vi "attribute_read_int64.vi"(5 "Repeated Capability":string, 7 "Attribute":T1={"Identifier"="", "Descriptive name"="", "Data Type"=enum."Integer 32", "Command"="", "Access"=2, "Range Table"="", "Read Callback"="", "Write Callback"="", "Range Callback"="", "Check Callback"="", "Rngtable Callback"="", "Coerce Callback"="", "Supported Models"="", "Instrument Options"="", "Repeated Capabilities"="", "Check Status Callback"="", "Index"=0, "Flag: OPC Wait"=FALSE, "Flag: Dont check status"=FALSE, "Flag: Cache Only"=FALSE} {"Access" items=["Read Only", "Write Only", "Read/Write"]}, 8 "error in":errorcluster, 11 "VISA resource name":refnum<visa-resource-name>) -> (0 "error out":errorcluster, 2 "int64 out":i64, 3 "VISA resource name out":refnum<visa-resource-name>)   [LabVIEW 2014, in "rszvl_rsidr_core.lvlib"]
uses:
  rszvl_rsidr_core.lvlib
  type_Attribute.ctl
  type_Attribute_Data_Type.ctl
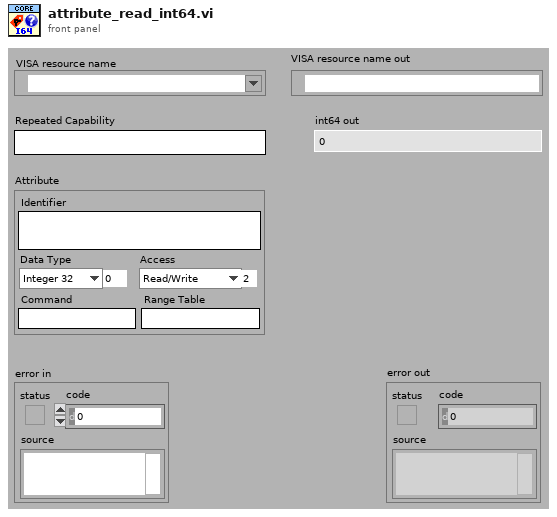
[diagram p1: front panel]
types:
  T1 = typedef "rszvl_rsidr_core.lvlib/type_Attribute.ctl" = cluster{"Identifier":string, "Descriptive name":string, "Data Type":T2, "Command":string, "Access":u16, "Range Table":string, "Read Callback":string, "Write Callback":string, "Range Callback":string, "Check Callback":string, "Rngtable Callback":string, "Coerce Callback":string, "Supported Models":string, "Instrument Options":string, "Repeated Capabilities":string, "Check Status Callback":string, "Index":i32, "Flag: OPC Wait":bool, "Flag: Dont check status":bool, "Flag: Cache Only":bool}
  T2 = typedef "rszvl_rsidr_core.lvlib/type_Attribute_Data_Type.ctl" = enum16{"Integer 32", "Double", "String", "Boolean", "None", "Integer 64"}
  T3 = typedef "rszvl_rsidr_core.lvlib/type_Session_Data.ctl" = cluster{"Instr type":string, "Instr type for err. msg.":string, "Installed Options":string[], "OPC Timeout":i32, "Query Instrument Status":bool, "Check Range":bool, "Check Options":bool, "Add LF to Write":bool, "Simulate":bool, "Logging":bool, "Logging params":variant, "Interface Type":enum16{"Unknown", "GPIB", "VXI", "GPIB_VXI", "ASRL", "PXI", "TCPIP", "USB", "SOCKET"}, "Fast Sweep":i32, "AdditionalFlags":i32, "WaitBeforeWrite":i32, "WaitBeforeRead":i32, "BinDataChunkSize":i64}
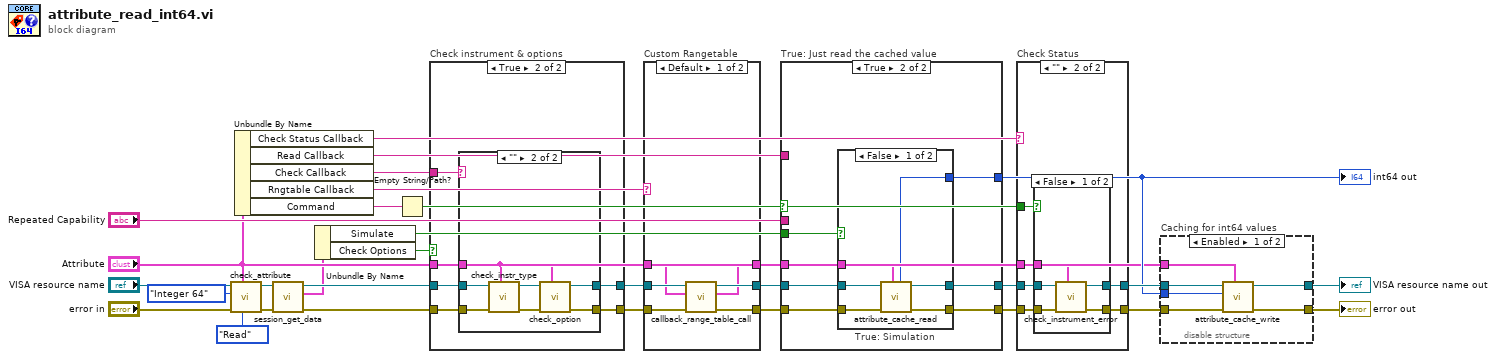
[diagram p0: block diagram]
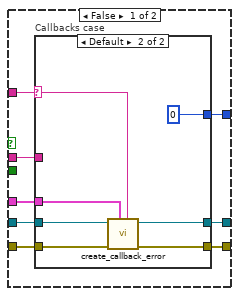
[diagram p2: hidden frame]
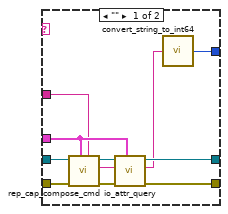
[diagram p3: hidden frame]
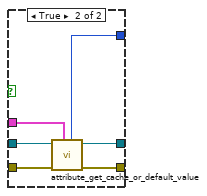
[diagram p4: hidden frame]
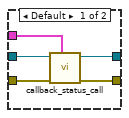
[diagram p6: hidden frame]
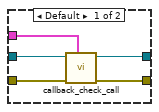
[diagram p9: hidden frame]
diagram:
  n1 = call "check_attribute.vi"("Access"=enum16{"Read", "Write"}."Read", "Attribute"="Attribute", "error in"="error in", "Data Type"=type_Attribute_Data_Type."Integer 64", "VISA resource name"="VISA resource name") -> ("error out"=w17:errorcluster, "VISA resource name out"=w18:refnum<visa-resource-name>)  [unwired: 5 in]
  n2 = Unbundle By Name("Attribute") -> ("Check Status Callback"=w19:string, "Read Callback"=w20:string, "Check Callback"=w9:string, "Rngtable Callback"=w10:string, "Command"=w5:string)
  n3 = call "session_get_data.vi"("error in"=w17, "VISA resource name"=w18) -> ("error out"=w3:errorcluster, "Session User Data out"=w1:T3, "VISA resource name out"=w16:refnum<visa-resource-name>)  [unwired: 7 in]
  n4 = Unbundle By Name(w1) -> ("Simulate"=w2:bool, "Check Options"=w15:bool)
  n5 = Empty String/Path?(string/path=w5) -> (empty?=w28:bool)
  n6 = case "Check instrument & options" shown="True" w15 {
    tunnel: [w33 w39] -> w14
    tunnel: [w32 w38] -> w13
    tunnel: w9 -> [_ w37]
    tunnel: w3 -> [w32 w36]
    tunnel: w16 -> [w33 w35]
    tunnel: "Attribute" -> [_ w34]
    frame False {
    }
    frame True {
      n7 = case shown="\"\"" w37 {
        tunnel: [w43 w49] -> w39
        tunnel: [w41 w48] -> w38
        tunnel: w36 -> [w42 w47]
        tunnel: w35 -> [w44 w46]
        tunnel: w34 -> [w40 w45]
        frame Default {
          n8 = call "callback_check_call.vi"("Attribute"=w40, "error in"=w42, "VISA resource name"=w44) -> ("error out"=w41:errorcluster, "VISA resource name out"=w43:refnum<visa-resource-name>)  [unwired: 7 in]
        }
        frame "" {
          n9 = call "check_instr_type.vi"("Attribute"=w45, "error in"=w47, "VISA resource name"=w46) -> ("error out"=w51:errorcluster, "VISA resource name out"=w50:refnum<visa-resource-name>)  [unwired: 6 in, 1 out]
          n10 = call "check_option.vi"("Attribute"=w45, "error in"=w51, "VISA resource name"=w50) -> ("error out"=w48:errorcluster, "VISA resource name out"=w49:refnum<visa-resource-name>)  [unwired: 7 in]
        }
      }
    }
  }
  n11 = case "Custom Rangetable" shown="Default" w10 {
    tunnel: w14 -> [w57 w60]
    tunnel: w13 -> [w54 w59]
    tunnel: [w56 w60] -> w12
    tunnel: [w55 w59] -> w11
    tunnel: "Attribute" -> [w53 w58]
    tunnel: [w52 w58] -> w8
    frame Default {
      n12 = call "callback_range_table_call.vi"("error in"=w54, "Attribute in"=w53, "VISA resource name"=w57) -> ("error out"=w55:errorcluster, "Attribute out"=w52:T1, "VISA resource name out"=w56:refnum<visa-resource-name>)  [unwired: 6 in]
    }
    frame "" {
    }
  }
  n13 = case "True: Just read the cached value" shown="True" w28 {
    tunnel: "Repeated Capability" -> [w68 _]
    tunnel: [w67 w91] -> w22
    tunnel: [w66 w90] -> w21
    tunnel: [w65 w88] -> w23
    tunnel: w20 -> [w64 _]
    tunnel: w12 -> [w63 w93]
    tunnel: w11 -> [w62 w92]
    tunnel: w8 -> [w61 w89]
    tunnel: w2 -> [_ w87]
    frame False {
      n14 = case "Callbacks case" shown="Default" w64 {
        selector: w64 -> [_ w80]
        tunnel: w63 -> [w79 w84]
        tunnel: w62 -> [w78 w85]
        tunnel: w68 -> [w72 _]
        tunnel: [w71 w82] -> w66
        tunnel: [w69 w83] -> w67
        tunnel: [w77 i64 0 ("int64 value out")] -> w65
        tunnel: w61 -> [w73 w81]
        frame "" {
          n15 = call "rep_cap_compose_cmd.vi"("Repeated Capability"=w72, "Attribute"=w73, "error in"=w78, "VISA resource name"=w79) -> ("error out"=w76:errorcluster, "Command out"=w74:string, "VISA resource name out"=w75:refnum<visa-resource-name>)  [unwired: 5 in]
          n16 = call "io_attr_query.vi"("Attribute"=w73, "error in"=w76, "write buffer"=w74, "VISA resource name"=w75) -> ("error out"=w69:errorcluster, "read buffer"=w70:string, "VISA resource name out"=w71:refnum<visa-resource-name>)  [unwired: 5 in]
          n17 = call "convert_string_to_int64.vi"("String in"=w70) -> ("int64 value out"=w77:i64)  [unwired: 4 in]
        }
        frame Default {
          n18 = call "create_callback_error.vi"("Callback Name"=w80, "Attribute"=w81, "error in"=w85, "VISA resource name"=w84) -> ("error out"=w83:errorcluster, "VISA resource name out"=w82:refnum<visa-resource-name>)  [unwired: 6 in]
        }
      }
    }
    frame True {
      n19 = case "True: Simulation" shown="False" w87 {
        tunnel: w92 -> [w99 w105]
        tunnel: w93 -> [w98 w104]
        tunnel: w89 -> [w97 w101]
        tunnel: [w96 w103] -> w91
        tunnel: [w95 w102] -> w90
        tunnel: [w94 w100] -> w88
        frame False {
          n20 = call "attribute_cache_read.vi"("Attribute"=w97, "error in"=w99, "VISA resource name"=w98) -> ("error out"=w96:errorcluster, "VISA resource name out"=w95:refnum<visa-resource-name>, "Integer 64 out"=w94:i64)  [unwired: 1 in, 5 out]
        }
        frame True {
          n21 = call "attribute_get_cache_or_default_value.vi"("Attribute"=w101, "error in"=w105, "VISA resource name"=w104) -> ("error out"=w103:errorcluster, "VISA resource name out"=w102:refnum<visa-resource-name>, "Integer 64 out"=w100:i64)  [unwired: 1 in, 5 out]
        }
      }
    }
  }
  "int64 out" <- w23
  n22 = case "Check Status" shown="\"\"" w19 {
    tunnel: w22 -> [w110 w114]
    tunnel: [w109 w113] -> w27
    tunnel: [w108 w115] -> w26
    tunnel: w21 -> [w107 w116]
    tunnel: w8 -> [w106 w112]
    tunnel: w28 -> [_ w111]
    frame Default {
      n23 = call "callback_status_call.vi"("Attribute"=w106, "error in"=w110, "VISA resource name"=w107) -> ("error out"=w109:errorcluster, "VISA resource name out"=w108:refnum<visa-resource-name>)  [unwired: 7 in]
    }
    frame "" {
      n24 = case shown="False" w111 {
        tunnel: w116 -> [w121 w123]
        tunnel: [w120 w123] -> w115
        tunnel: w114 -> [w119 w122]
        tunnel: [w118 w122] -> w113
        tunnel: w112 -> [w117 _]
        frame False {
          n25 = call "check_instrument_error.vi"("Attribute"=w117, "error in"=w119, "VISA resource name"=w121) -> ("error out"=w118:errorcluster, "VISA resource name out"=w120:refnum<visa-resource-name>)  [unwired: 7 in]
        }
        frame True {
        }
      }
    }
  }
  n26 = disable-structure "Caching for int64 values" shown="Enabled" {
    disable-tunnel: [w129 w131] -> w25
    disable-tunnel: [w128 w130] -> w24
    disable-tunnel: w27 -> [w127 w130]
    disable-tunnel: w26 -> [w126 w131]
    disable-tunnel: w23 -> [w125 _]
    disable-tunnel: "Attribute" -> [w124 _]
    frame Enabled {
      n27 = call "attribute_cache_write.vi"("Attribute"=w124, "error in"=w127, "Value in"=w125, "VISA resource name"=w126) -> ("error out"=w128:errorcluster, "VISA resource name out"=w129:refnum<visa-resource-name>)  [unwired: 6 in]
    }
    frame Disabled {
    }
  }
  "error out" <- w24
  "VISA resource name out" <- w25
